vi "Save Notebook Rich Text Box.vi"(6 "Backup?":bool, 7 "Default Notebook File Name (Notebook)":string="Notebook", 8 "Error In":errorcluster, 9 "Dialog (F)":bool, 10 "File Path Control":path, 11 ".NET Refnum in":refnum<k24>) -> (0 "Error Out":errorcluster, 1 "cancelled":bool, 2 "File Path out":path, 3 "Rtf Content":string)   [LabVIEW 2021, in "Notebook.lvlib"]
uses:
  Notebook.lvlib
  System.Windows.Forms
  Rich Text Box/Rich Text Box.lvlib
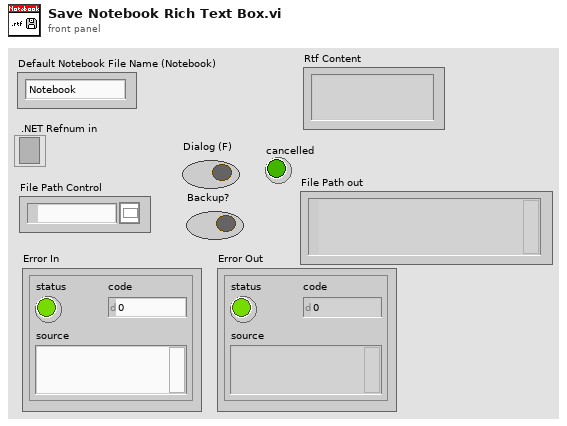
[diagram p1: front panel]
types:
  T1 = typedef "Rich Text Box.lvlib/Text Formatting.ctl" = cluster{"Font":string, "Text Color":T2, "Text Background Color":T2, "Text Style":enum16{"Regular", "Bold", "Italic", "Underline", "Strikeout"}, "Font Size (Points)":dbl, "Text Alignment":i32}
  T2 = typedef "Rich Text Box.lvlib/Text Colors.ctl" = enum16{"Unchanged", "Black", "Blue", "Brown", "Gray", "Green", "Orange", "Pink", "Red", "White"}
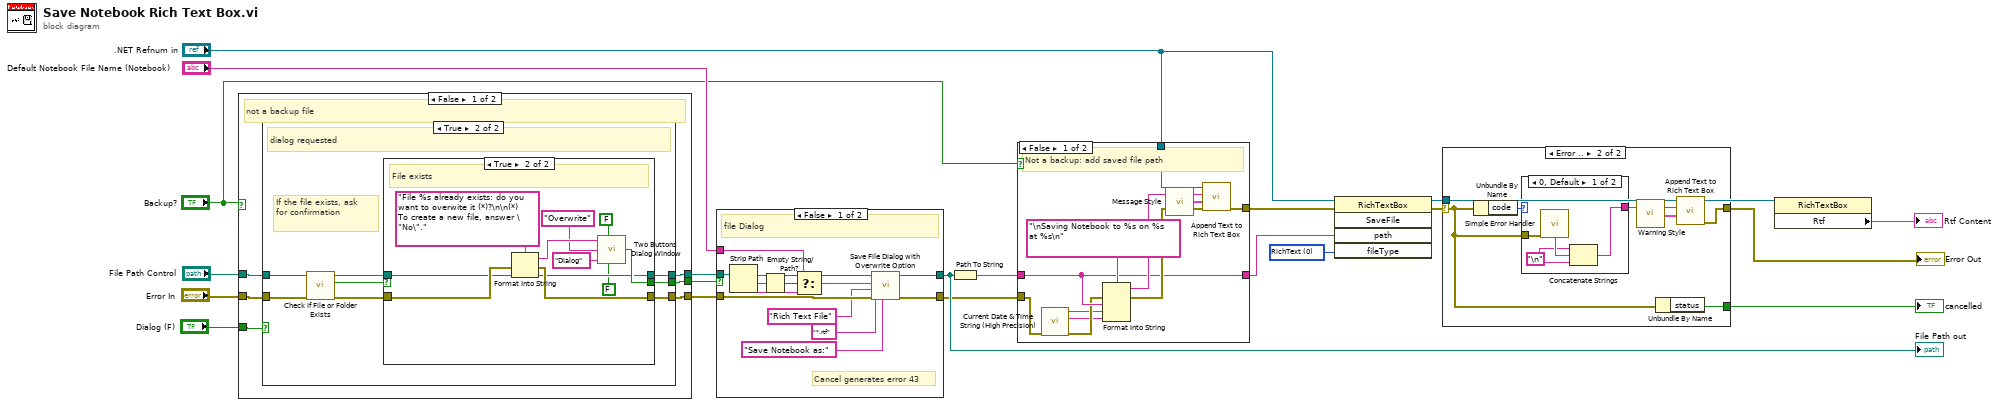
[diagram p0: block diagram]
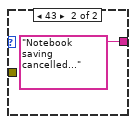
[diagram p4: hidden frame]
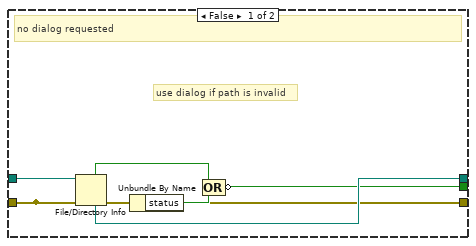
[diagram p6: hidden frame]
diagram:
  w19 = 0 items=["RichText", "PlainText", "RichNoOleObjs", "TextTextOleObjs", "UnicodePlainText"] ("fileType")
  n1 = case shown="False" "Backup?" {
    selector: "Backup?" -> [_ w57]
    tunnel: [w24 w56] -> w18
    tunnel: [w26 w55] -> w17
    tunnel: [w25 w57] -> w16
    tunnel: "Dialog (F)" -> [w21 _]
    tunnel: "File Path Control" -> [w23 w56]
    tunnel: "Error In" -> [w22 w55]
    frame False {
      # "not a backup file"
      n2 = case shown="True" w21 {
        tunnel: [w27 w41] -> w26
        tunnel: [w28 w40] -> w25
        tunnel: [w32 w39] -> w24
        tunnel: w23 -> [w33 w38]
        tunnel: w22 -> [w27 w37]
        frame False {
          # "use dialog if path is invalid"
          # "no dialog requested"
          n3 = File/Directory Info(path=w33, error in=w27) -> (directory=w29:bool, error out=w31:errorcluster, resolved path=w32:path)  [unwired: 4 out]
          n4 = Unbundle By Name(w31) -> ("status"=w30:bool)
          n5 = Compound Arithmetic op=OR(w29, w30) -> (invert w28:bool)
        }
        frame True {
          # "If the file exists, ask for confirmation"
          # "dialog requested"
          n6 = call <vilib>:"Check if File or Folder Exists.vi"("error in (no error)"=w37, "path"=w38) -> ("error out"=w36:errorcluster, "file or folder exists?"=w34:bool, "dup path"=w35:path)  [unwired: 7 in]
          n7 = case shown="True" w34 {
            selector: w34 -> [w42 _]
            tunnel: w36 -> [w43 w52]
            tunnel: [w43 w51] -> w41
            tunnel: [w42 w48] -> w40
            tunnel: w35 -> [w44 w47]
            tunnel: [w44 w47] -> w39
            frame False {
              # "File does not exist"
            }
            frame True {
              # "File exists"
              n8 = Format Into String(format string="File %s already exists: do you want to overwite it (*)?\n\n(*) To create a new file, answer \"No\".", error in=w52, w47) -> (resulting string=w53:string, error out=w51:errorcluster)  [unwired: 1 in]
              n9 = call "Two Buttons Dialog Window.vi"("Message"=w53, "Return =  OK (T)"=FALSE, "OK Button Text"="Overwrite" ("T button name (\"OK\")"), "Cancel Button Text"="Dialog" ("F button name (\"Cancel\")"), "ESC =  Cancel (T)"=FALSE) -> ("OK?"=w48:bool)  [unwired: 4 in]
            }
          }
        }
      }
    }
    frame True {
      # "backup: no dialog"
    }
  }
  n10 = case shown="False" w16 {
    tunnel: [w68 w70] -> w20
    tunnel: [w67 w71] -> w6
    tunnel: w18 -> [w66 w70]
    tunnel: w17 -> [w65 w71]
    tunnel: "Default Notebook File Name (Notebook)" -> [w58 _]
    frame False {
      # "Cancel generates error 43"
      # "file Dialog"
      n11 = Strip Path(path=w66) -> (stripped path=w64:path, name=w59:string)
      n12 = Empty String/Path?(string/path=w59) -> (empty?=w61:bool)
      n13 = Select(t=w58, s=w61, f=w59) -> (s? t:f=w60:string)
      n14 = call "Save File Dialog with Overwrite Option.vi"("prompt"="Save Notebook as:", "Default Name"=w60, "error in (no error)"=w65, "pattern label"="Rich Text File", "pattern (all files)"="*.rtf" ("pattern label"), "Starting Folder"=w64) -> ("error out"=w67:errorcluster, "selected path"=w68:path)  [unwired: 2 in, 2 out]
    }
    frame True {
      # "no dialog needed"
    }
  }
  "File Path out" <- w20
  n15 = Path To String(path=w20) -> (string=w2:string)
  n16 = case shown="False" "Backup?" {
    tunnel: ".NET Refnum in" -> [w82 _]
    tunnel: [w81 w84] -> w10
    tunnel: w6 -> [w75 w84]
    tunnel: w2 -> [w76 w83]
    tunnel: [w76 w83] -> w3
    frame False {
      # "Not a backup: add saved file path"
      n17 = call "Current Date & Time String (High Precision).vi"("Error In"=w75) -> ("Error Out"=w74:errorcluster, "time string"=w72:string, "date string"=w73:string)  [unwired: 7 in, 1 out]
      n18 = Format Into String(format string="\nSaving Notebook to %s on %s at %s\n", error in=w74, w76, w73, w72) -> (resulting string=w79:string, error out=w80:errorcluster)  [unwired: 1 in]
      n19 = call "Message Style.vi"() -> ("Message Formatting"=w77:T1)
      n20 = call "Append Text to Rich Text Box.vi"("error in (no error)"=w80, "Text Formatting"=w77, "String"=w79, ".NET Refnum in"=w82) -> ("Error Out"=w81:errorcluster)  [unwired: 6 in, 1 out]
    }
    frame True {
      # "backup file"
    }
  }
  n21 = invoke class="RichTextBox" method="SaveFile"(reference=".NET Refnum in", error in=w10, "path"=w3, "fileType"=w19) -> (reference out=w7:refnum<k24>, error out=w9:errorcluster)  [unwired: 1 in, 3 out]
  n22 = case shown="Error .." w9 {
    selector: w9 -> [w85 w86]
    tunnel: [w85 w90] -> w1
    tunnel: [_ w92] -> w8
    tunnel: w7 -> [_ w91]
    frame No Error {
    }
    frame Error {
      n23 = Unbundle By Name(w86) -> ("code"=w88:i32)
      n24 = case shown="0, Default" w88 {
        tunnel: [w94 "Notebook saving cancelled..." ("String")] -> w87
        tunnel: w86 -> [w96 _]
        frame 0, Default {
          w93 = "\n"
          n25 = call <vilib>:"Simple Error Handler.vi"("error in (no error)"=w96) -> ("message"=w95:string)  [unwired: 4 in, 4 out]
          n26 = Concatenate Strings(w93, w95, w93) -> (w94:string)
        }
        frame 43 {
        }
      }
      n27 = call "Warning Style.vi"() -> ("Error Formatting"=w89:T1)
      n28 = Unbundle By Name(w86) -> ("status"=w92:bool)
      n29 = call "Append Text to Rich Text Box.vi"("Text Formatting"=w89, "String"=w87, ".NET Refnum in"=w91) -> ("Error Out"=w90:errorcluster)  [unwired: 7 in, 1 out]
    }
  }
  "Error Out" <- w1
  "cancelled" <- w8
  n30 = property class="RichTextBox"(reference=w7) -> ("Rtf"=→"Rtf Content":string)  [unwired: 1 in, 2 out]
